vi "T90 Zustandsautomat.vi"(0 "Aktion":T1, 11 "error in (no error)":errorcluster caption="Fehler (Eingang, kein Fehler)") -> (4 "Aktion":T1, 8 "Aufschaltzeit":dbl, 10 "Status":string, 15 "error out":errorcluster caption="Fehler (Ausgang)")   [LabVIEW 2020, in "EPA 1065.lvlib" / "T90 Test 1065-308.lvlib"]
uses:
  T90 Test 1065-308.lvlib
  Aktion T90 Zustandsautomat.ctl
  Aktion FGV Datenmanagment.ctl
  Sprachverwaltung/FGV Aktion Tabelle zerlegen.ctl
  Aktion FGV T90.ctl
  Seiten/CalGas Aufschaltung/FGV CalGas Aktionen.ctl
  Seiten/CalGas Aufschaltung/Auswahl Aufschaltpunkt.ctl
  Funktionstasten/Zustaende.ctl
  Funktionstasten/Funktionstasten-Aktion.ctl
  PNS/Aktionen FGV Grenzwerte.ctl
  Sprachverwaltung/Sprachverwaltung.lvlib
  Funktionstasten/Funktionstasten.lvlib
  Allgemein/allgemeine Sub-VIs.lvlib
  Seiten/CalGas Aufschaltung/CalGas Aufschaltung.lvlib
  PNS/PNS.lvlib
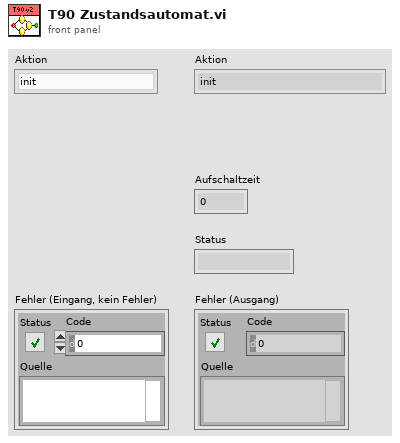
[diagram p1: front panel]
types:
  T1 = typedef "EPA 1065.lvlib/T90 Test 1065-308.lvlib/Aktion T90 Zustandsautomat.ctl" = enum16{"init", "start", "CG aufschalten", "Aufschaltzeit einhalten", "Peak ermitteln", "spülen", "CG Sequenz T10", "CG Sequenz T90", "CG halten", "N2 Sequenz T90", "N2 Sequenz T10", "N2 halten", "Auswerten", "abbrechen", "Störung", "fertig"}
  T2 = typedef "EPA 1065.lvlib/T90 Test 1065-308.lvlib/Aktion FGV Datenmanagment.ctl" = enum16{"init", "lesen", "Istwerte schreiben", "höchsten Peak setzen", "Auswerten", "Grenzen setzen", "Sollwert ändern", "Rise T10", "Rise T90", "Fall T90", "Fall T10", "Bit löschen", "Umschaltzeitpunkt"}
  T3 = typedef "Sprachverwaltung.lvlib/FGV Aktion Tabelle zerlegen.ctl" = enum16{"laden", "vereinzeln", "speichern"}
  T4 = typedef "CalGas Aufschaltung.lvlib/FGV CalGas Aktionen.ctl" = enum16{"lesen", "Analysator Auswahl", "Def.CalGas", "Aufschaltung CalGas", "laden", "speichern", "KAL extrahieren"}
  T5 = typedef "EPA 1065.lvlib/T90 Test 1065-308.lvlib/Aktion FGV T90.ctl" = enum16{"lesen", "Konfig Daten", "speichern", "laden", "T90 aktiv", "T90 inaktiv", "Ext. Ventil aktivieren", "Ext. Ventil deaktivieren", "N2 spülen aktiv", "N2 spülen inaktiv", "Ergebnis Textfile"}
  T6 = typedef "CalGas Aufschaltung.lvlib/Auswahl Aufschaltpunkt.ctl" = enum16{"über Filterblock", "Analysator direkt", "über PNS", "Entnahme", "Gasdivider"}
  T7 = typedef "Funktionstasten.lvlib/Funktionstasten-Aktion.ctl" = enum16{"Initialisieren", "Zustand setzen", "Taste gedrückt", "Fehler speichern", "Lesen", "Manuell", "Remote", "Bitparallel", "Samplepoint", "Zeit Prüfen", "reset Umschalten"}
  T8 = typedef "Funktionstasten.lvlib/Zustaende.ctl" = enum16{"Standby", "Pause", "Eco", "Messen", "Kalibrieren", "Spülen Filter", "Spülen Leitung", "Umgebungsluft", "0-Gas", "Cal-Gas", "CG zu PNS", "-------------", "Init 1", "Init 2", "Init 3", "Init 4", "Messen vorbereiten", "Messen durchführen", "Exit"}
  T9 = typedef "PNS.lvlib/Aktionen FGV Grenzwerte.ctl" = enum16{"lesen", "Grenzw. schreiben", "Anweisungscode", "IP-Adresse", "laden", "speichern", "Anweisungscode vorgeben"}
  T10 = typedef "CalGas Aufschaltung.lvlib/Aufschaltung CalGas.ctl" = cluster{"Kalibriergas":T11, "Aufschaltpunkt":T6, "Analysator":T12}
  T11 = typedef "Auswahlfeld.ctl" = u16
  T12 = typedef "CalGas Aufschaltung.lvlib/Auswahl Analysator.ctl" = enum16{"FT-IR", "FID", "PMA", "PMA/FID/FT-IR"}
  T13 = typedef "EPA 1065.lvlib/T90 Test 1065-308.lvlib/T90 Konfig Daten.ctl" = cluster{"Bearbeiter:":string, "Komponente:":u16, "Gasflaschen Nr.:":string, "Accuracy":dbl, "Sollwert":dbl, "Modus":T14, "Abschaltzeit:":dbl, "Abweichung:":dbl, "Pfad:":path, "Textname:":string, "CG Aufschaltzeit:":dbl, "Einheit":string, "N2 Aufschaltzeit:":dbl, "Analysator":T15, "Gasflasche":T16, "Konfig Gasflasche":T17, "Frequency:":T18}
  T14 = typedef "EPA 1065.lvlib/T90 Test 1065-308.lvlib/Modus.ctl" = u16
  T15 = typedef "System Einstellungen V2.lvlib/Analysatoren.ctl" = string
  T16 = typedef "System Einstellungen V2.lvlib/Gasflasche Auswahl.ctl" = u16
  T17 = typedef "System Einstellungen V2.lvlib/Konfig Gasflasche.ctl" = bool
  T18 = typedef "EPA 1065.lvlib/T90 Test 1065-308.lvlib/Frequenz.ctl" = u16
  T19 = typedef "EPA 1065.lvlib/T90 Test 1065-308.lvlib/Datencluster.ctl" = cluster{"Höchster Peak":T20, "T10 Grenzwert":T20, "T90 Grenzwert":T20, "Rise Times":dbl[], "Fall Times":dbl[], "RiseTime gemittelt":T20, "FallTime gemittelt":T20, "Zeitstempel":timestamp[], "Rise T10":bool, "Rise T90":bool, "Fall T10":bool, "Fall T90":bool, "RiseTime >5":bool, "Falltime >5":bool, "RiseTime <10":bool, "Falltime <10":bool, "T0-T90":dbl[], "T100-T10":dbl[]}
  T20 = typedef "Zahlen-Eingabefeld.ctl" = sgl
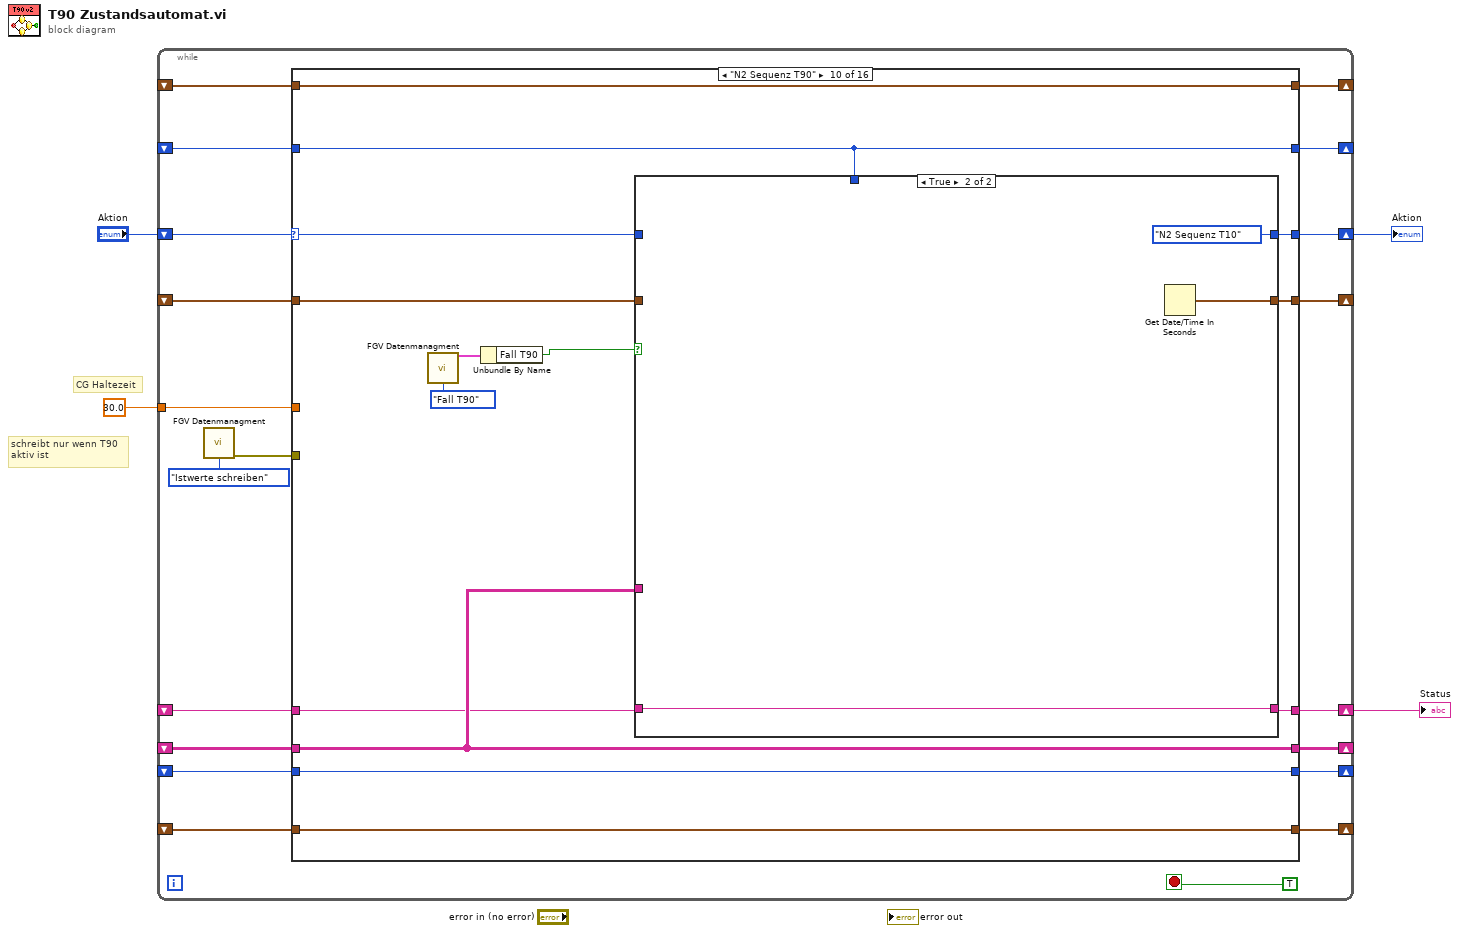
[diagram p0: block diagram]
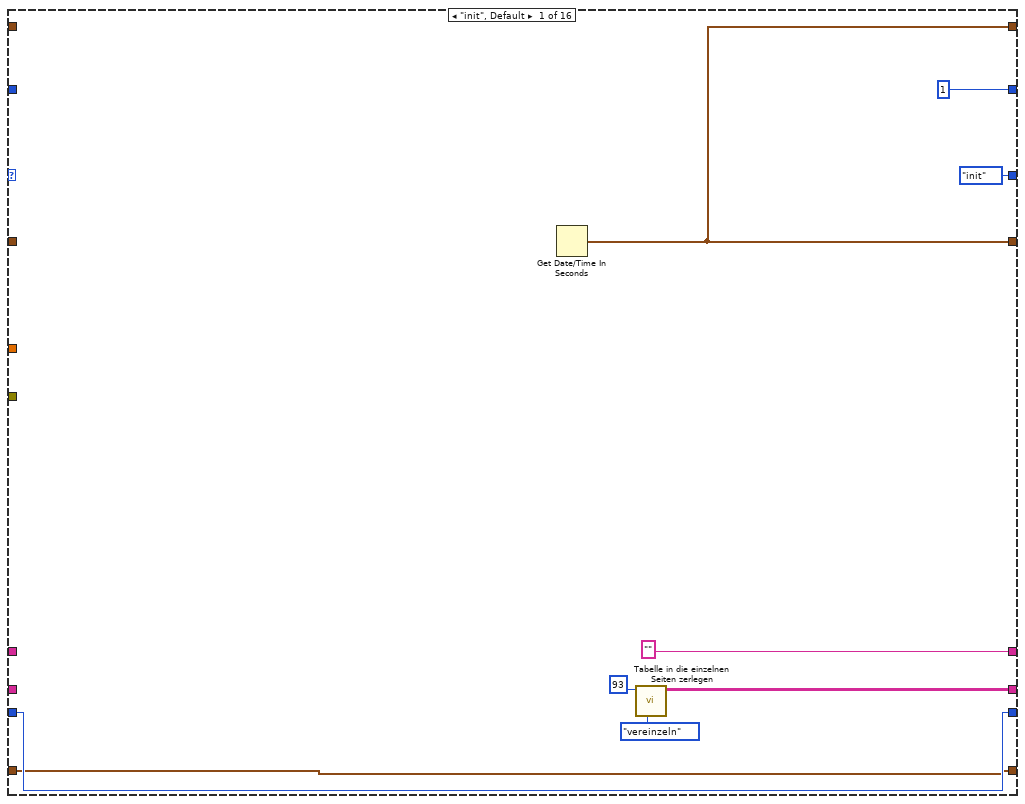
[diagram p2: hidden frame]
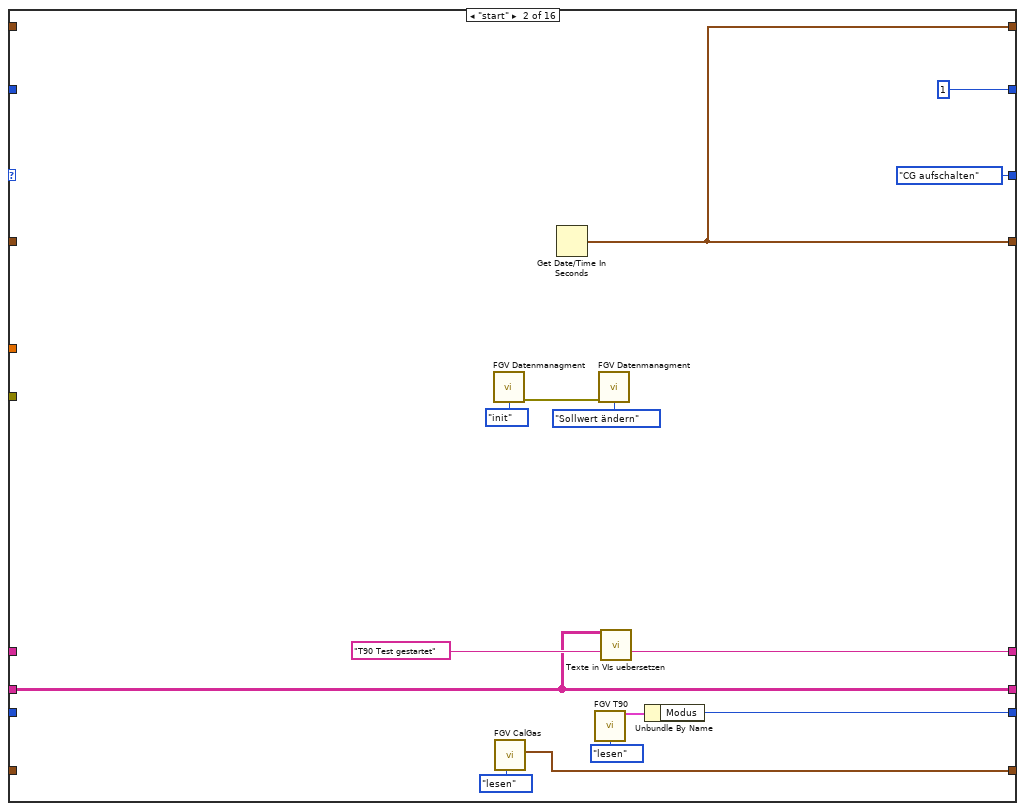
[diagram p3: hidden frame]
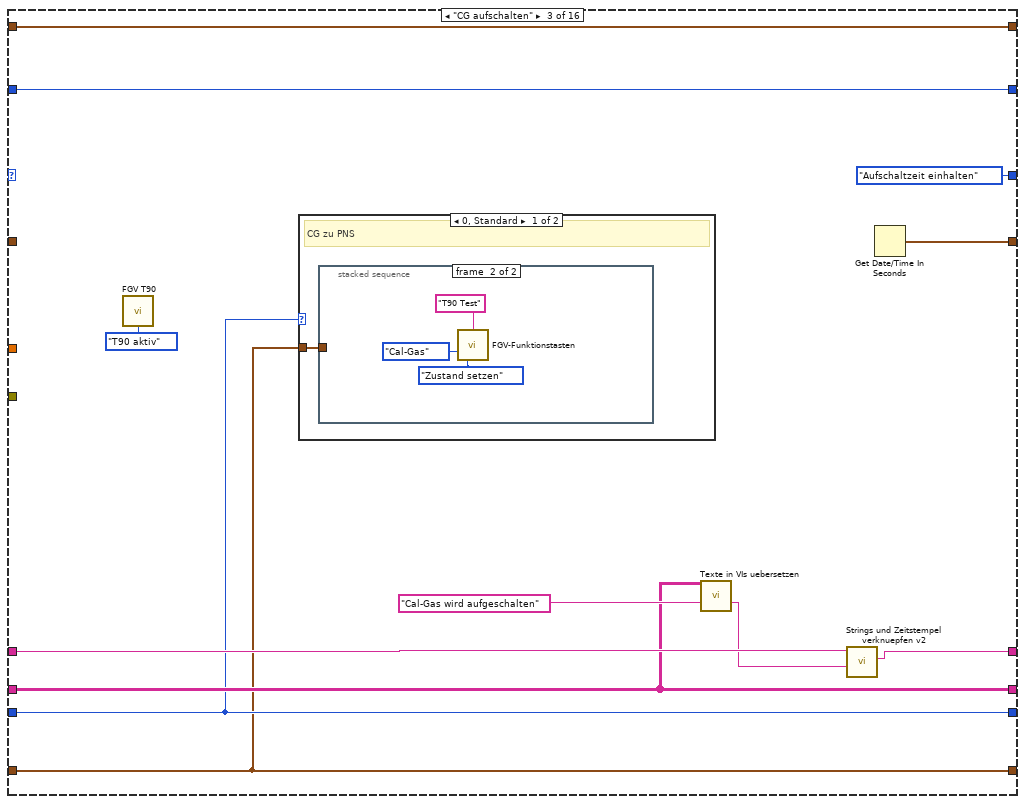
[diagram p4: hidden frame]
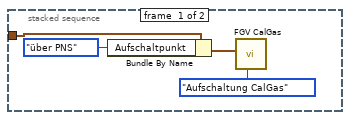
[diagram p5: hidden frame]
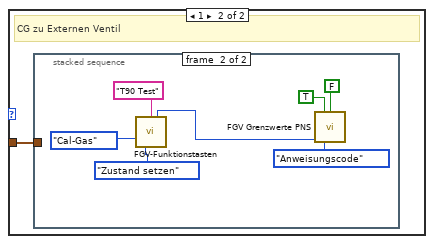
[diagram p6: hidden frame]
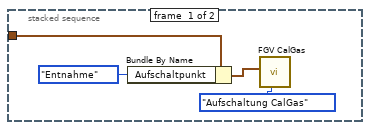
[diagram p7: hidden frame]
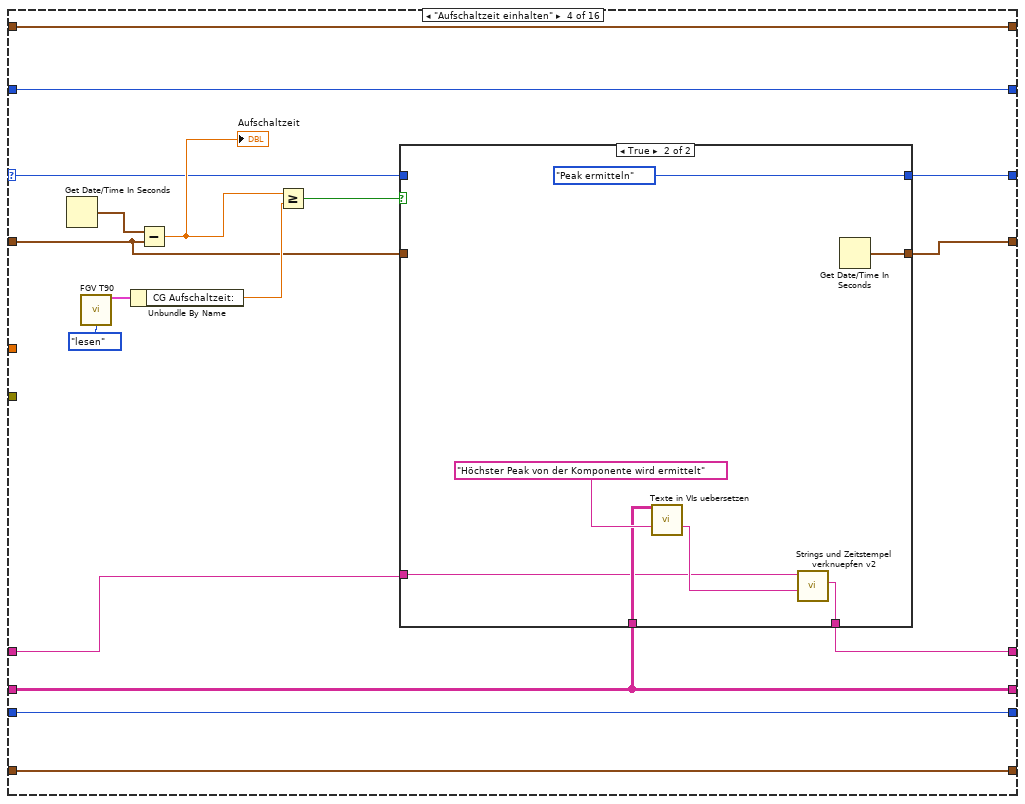
[diagram p8: hidden frame]
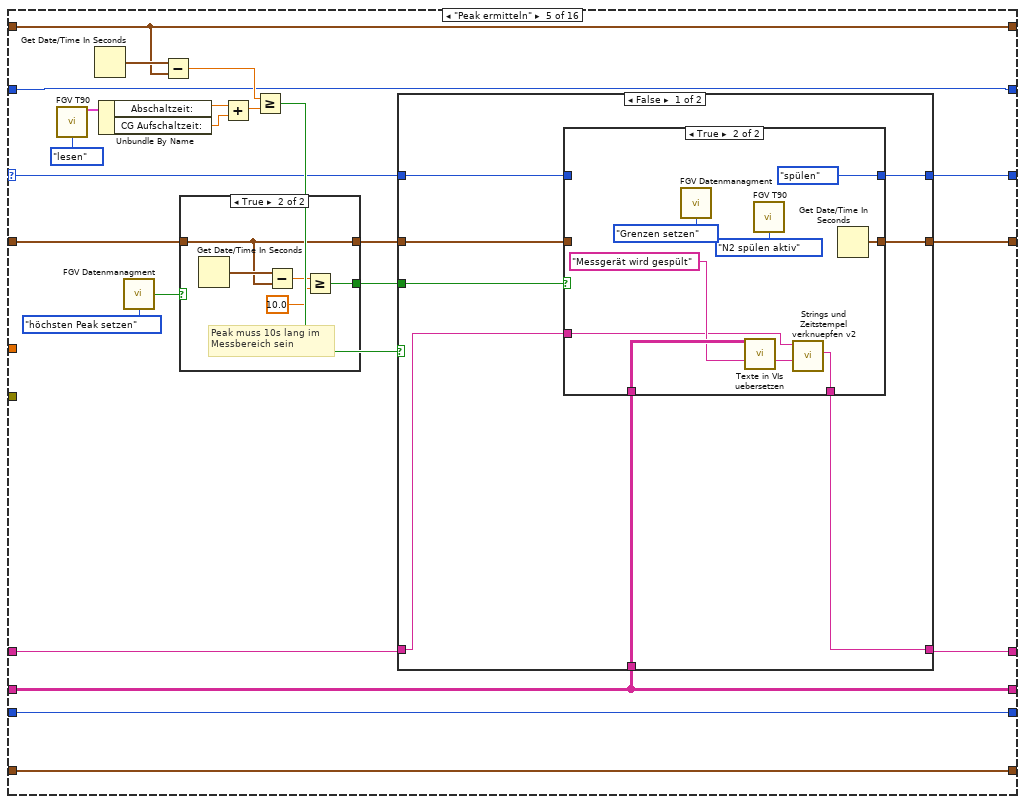
[diagram p10: hidden frame]
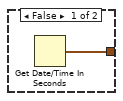
[diagram p11: hidden frame]
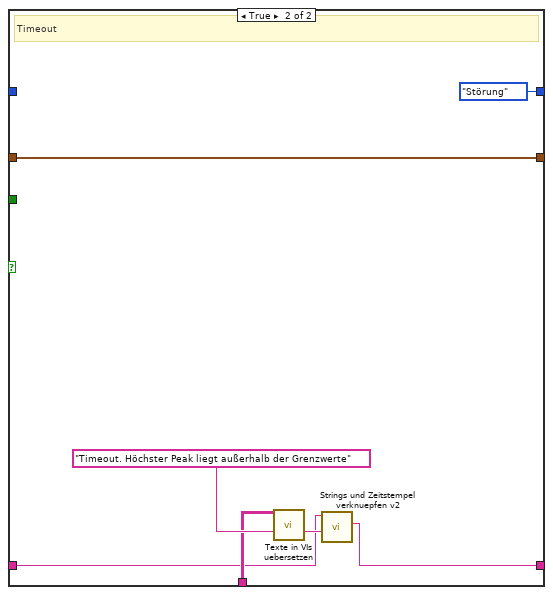
[diagram p13: hidden frame]
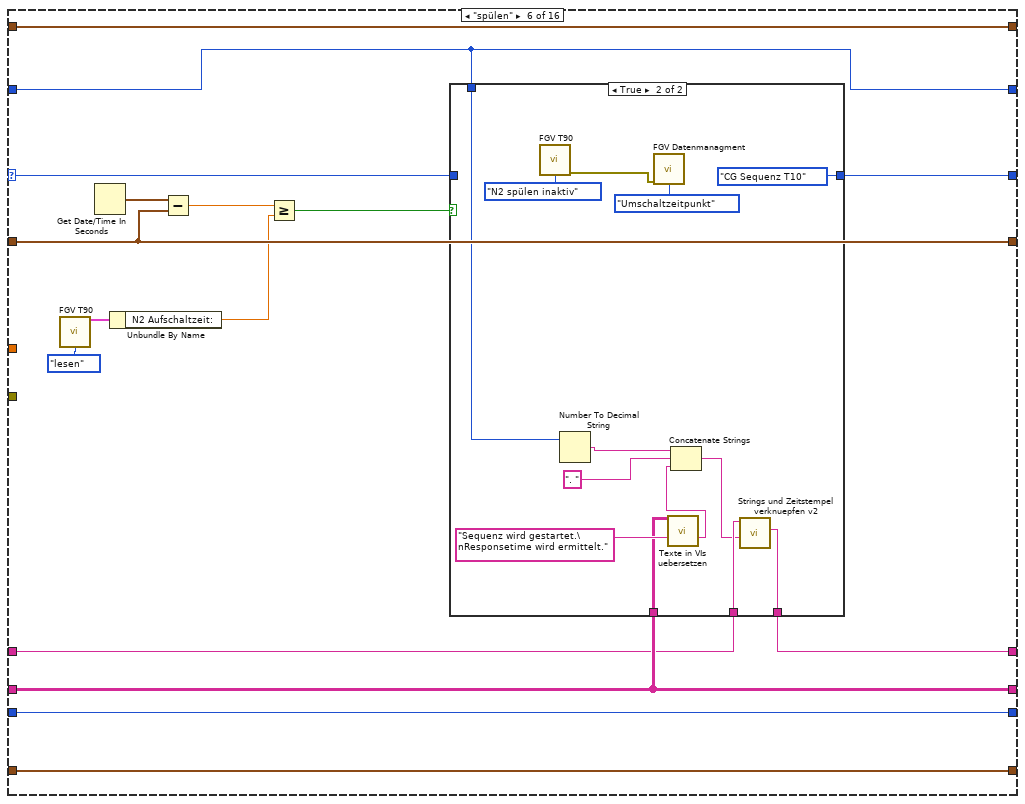
[diagram p14: hidden frame]
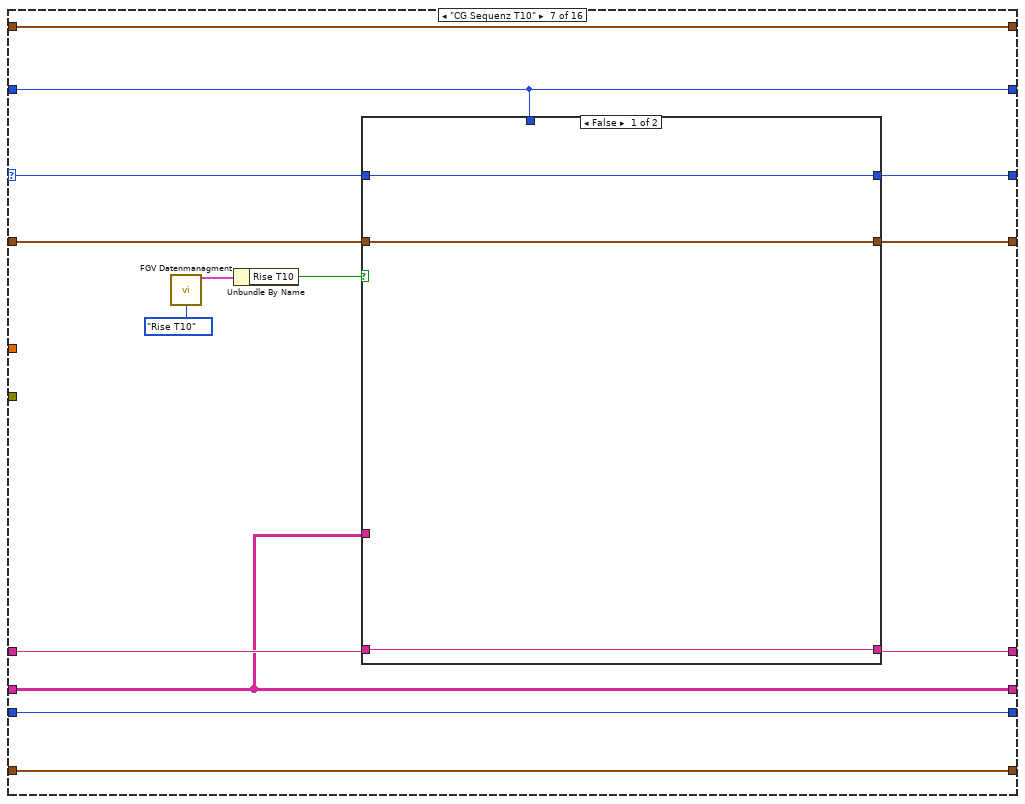
[diagram p16: hidden frame]
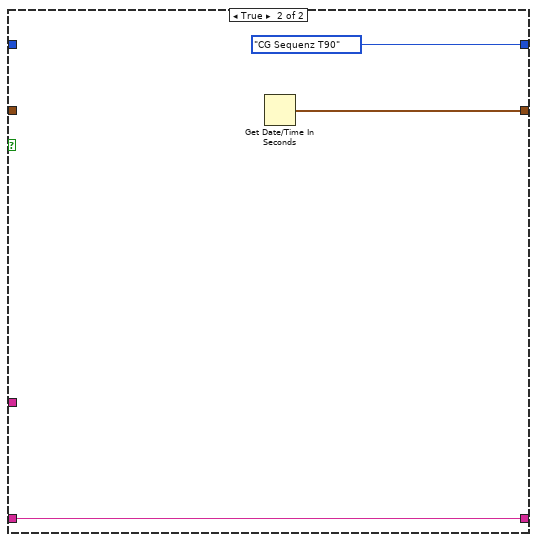
[diagram p17: hidden frame]
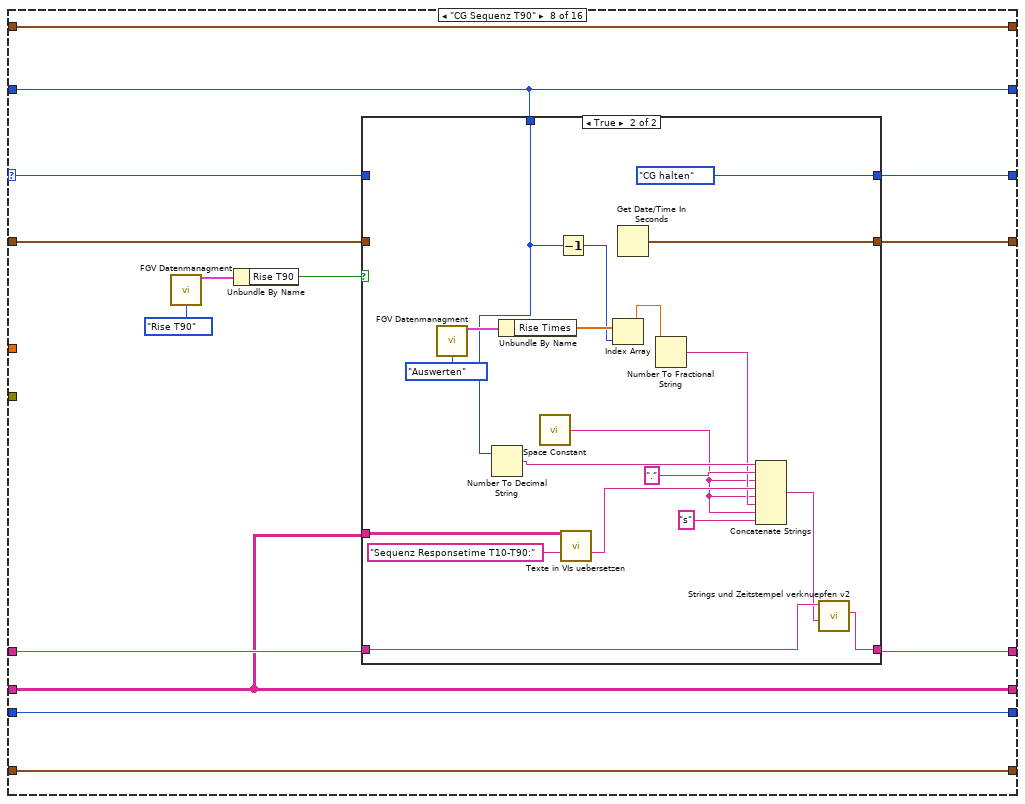
[diagram p18: hidden frame]
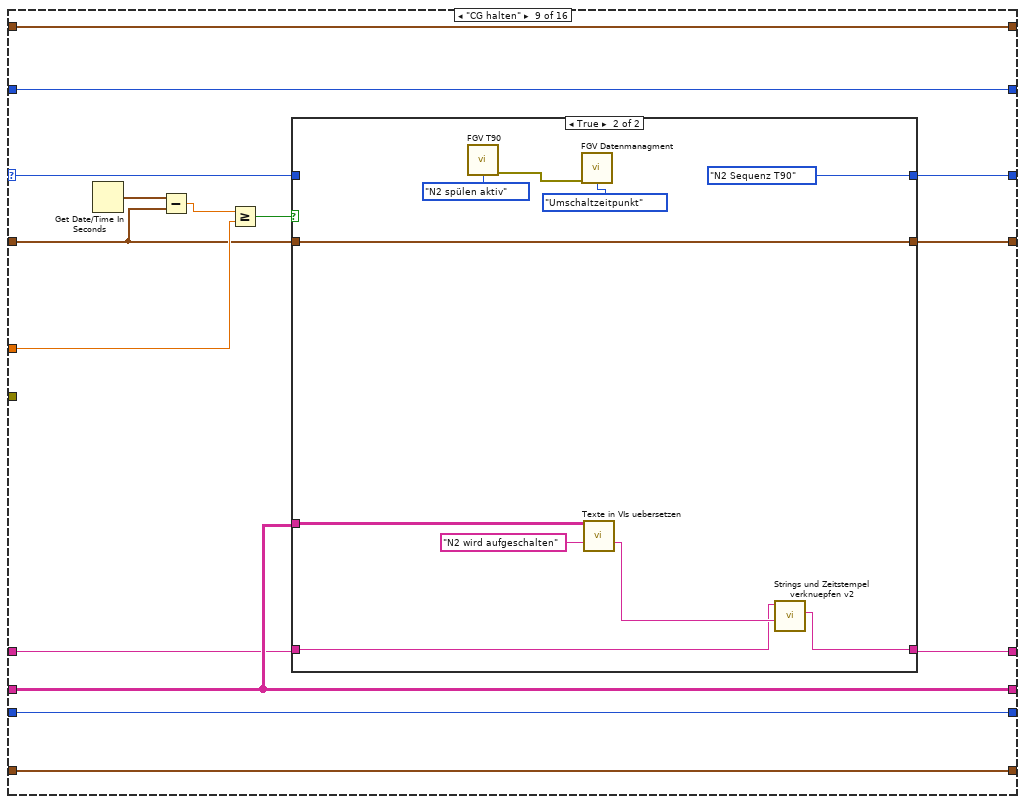
[diagram p20: hidden frame]
diagram:
  # "schreibt nur wenn T90\naktiv ist"
  # "CG Haltezeit"
  n1 = while {
    shift-right: [w23] -> w1
    shift-left: "Aktion" -> [w22]
    shift-right: [w21] -> _
    shift-left: _ -> [w20]
    shift-right: [w19] -> w3
    shift-left: _ -> [w17]
    shift-right: [w16] -> _
    shift-left: _ -> [w18]
    tunnel: 30.0 ("x-y") -> [w15]
    shift-right: [w14] -> _
    shift-left: _ -> [w13]
    shift-right: [w11] -> _
    shift-left: _ -> [w12]
    shift-right: [w8] -> _
    shift-left: _ -> [w7]
    shift-right: [w6] -> _
    shift-left: _ -> [w5]
    stop <- TRUE stop-if-true
    n2 = call "FGV Datenmanagment.vi"("Aktion"=Aktion_FGV_Datenmanagment."Istwerte schreiben") -> ("error out"=w9:errorcluster)  [unwired: 7 in, 7 out]
    n3 = case shown="\"N2 Sequenz T90\"" w22 {
      selector: w22 -> [_ _ _ w89 w122 w174 w205 w225 w260 w289 w309 w349 _ _ _ _]
      tunnel: [Aktion_T90_Zustandsautomat."init" ("Aktion") Aktion_T90_Zustandsautomat."CG aufschalten" ("Aktion") Aktion_T90_Zustandsautomat."Aufschaltzeit einhalten" ("Aktion") w91 w123 w173 w204 w224 w259 w288 w308 w348 Aktion_T90_Zustandsautomat."fertig" ("Aktion") Aktion_T90_Zustandsautomat."fertig" ("Aktion") Aktion_T90_Zustandsautomat."fertig" ("Aktion") Aktion_T90_Zustandsautomat."fertig" ("Aktion")] -> w23
      tunnel: [w27 w44 w59 w82 w117 w177 w203 w223 w257 w287 w307 w346 w387 w406 w418 w426] -> w16
      tunnel: [w30 w40 w52 w87 w120 w172 w199 w219 w255 w285 w305 w343 w394 w404 w422 w430] -> w21
      tunnel: w20 -> [_ w40 w52 w87 w120 w172 w199 w219 w255 w285 w305 w343 w394 w404 w422 w430]
      tunnel: ["" w34 w55 w86 w118 w170 w200 w220 w253 w284 w304 w341 w385 w395 w416 w425] -> w19
      tunnel: w18 -> [_ _ _ w83 w111 w177 w202 w222 w258 w286 w306 w347 w387 w406 w418 w426]
      tunnel: w17 -> [_ _ w56 w85 w119 w171 w201 w221 w254 w283 w303 w342 w385 _ w416 w425]
      tunnel: w15 -> [_ _ _ _ _ _ _ _ w262 _ _ _ _ _ _ _]
      tunnel: [1 1 w57 w88 w121 w169 w198 w218 w256 w282 w302 w344 w393 w408 w419 w429] -> w14
      tunnel: w13 -> [_ _ w57 w88 w121 w169 w198 w218 w256 w282 w302 w345 w393 w408 w419 w429]
      tunnel: [w27 w44 w51 w84 w116 w168 w197 w217 w252 w281 w301 w340 w384 w403 w417 w428] -> w11
      tunnel: w12 -> [_ _ w51 w84 w116 w168 w197 w217 w252 w281 w301 w340 w384 w403 w417 w428]
      tunnel: w9 -> [_ _ _ _ _ _ _ _ _ _ _ _ _ _ _ _]
      tunnel: [w26 w37 w49 w81 w108 w167 w195 w215 w251 w279 w299 w339 w383 w398 w411 w424] -> w8
      tunnel: w7 -> [w26 _ w49 w81 w108 w167 w195 w215 w251 w279 w299 w339 w383 w398 w411 w424]
      tunnel: [w25 w35 w48 w80 w107 w166 w194 w214 w250 w278 w298 w338 w381 w396 w409 w423] -> w6
      tunnel: w5 -> [w25 _ w48 w80 w107 w166 w194 w214 w250 w278 w298 w338 w381 w396 w409 w423]
      frame "init", Default {
        n4 = Get Date/Time In Seconds() -> (seconds since 1Jan1904=w27:timestamp)
        n5 = call "Tabelle in die einzelnen Seiten zerlegen.vi"("Aktion"=FGV_Aktion_Tabelle_zerlegen."vereinzeln", "Index (Seite)"=93) -> ("Sprachliste"=w30:string[][])  [unwired: 7 in, 2 out]
      }
      frame "start" {
        n6 = call "FGV Datenmanagment.vi"("Aktion"=Aktion_FGV_Datenmanagment."init") -> ("error out"=w42:errorcluster)  [unwired: 7 in, 7 out]
        n7 = call "FGV CalGas.vi"("Aktionen"=FGV_CalGas_Aktionen."lesen") -> ("Aufschaltung CalGas"=w35:T10)  [unwired: 6 in, 4 out]
        n8 = Get Date/Time In Seconds() -> (seconds since 1Jan1904=w44:timestamp)
        n9 = call "FGV T90.vi"("Aktion"=Aktion_FGV_T90."lesen") -> ("T90 Konfig Daten"=w38:T13)  [unwired: 9 in, 5 out]
        n10 = call "FGV Datenmanagment.vi"("error in (no error)"=w42, "Aktion"=Aktion_FGV_Datenmanagment."Sollwert ändern") -> ()  [unwired: 6 in, 8 out]
        n11 = call "Texte in VIs uebersetzen.vi"("Sprachliste"=w40, "String zum Übersetzen"="T90 Test gestartet" ("String 1 hinzufügen")) -> ("String zum Übersetzen"=w34:string)  [unwired: 9 in, 4 out]
        n12 = Unbundle By Name(w38) -> ("Modus"=w37:T14)
      }
      frame "CG aufschalten" {
        n13 = call "FGV T90.vi"("Aktion"=Aktion_FGV_T90."T90 aktiv") -> ()  [unwired: 9 in, 6 out]
        n14 = case shown="0, Standard" w49 {
          tunnel: w48 -> [w60 w68]
          frame 0, Default {
            # "CG zu PNS"
            n15 = stacked-sequence {
              tunnel: w60 -> [w63 _]
              frame #0 {
                n16 = Bundle By Name(cluster=w63, "Aufschaltpunkt"=Auswahl_Aufschaltpunkt."über PNS") -> (w61:T10)
                n17 = call "FGV CalGas.vi"("Aktionen"=FGV_CalGas_Aktionen."Aufschaltung CalGas", "Aufschaltung CalGas"=w61) -> ()  [unwired: 5 in, 5 out]
              }
              frame #1 {
                n18 = call "FGV-Funktionstasten.vi"("Herkunft"="T90 Test", "Zustand"=Zustaende."Cal-Gas", "Aktion"=Funktionstasten-Aktion."Zustand setzen") -> ()  [unwired: 5 in, 8 out]
              }
            }
          }
          frame 1 {
            # "CG zu Externen Ventil"
            n19 = stacked-sequence {
              tunnel: w68 -> [w71 _]
              frame #0 {
                n20 = Bundle By Name(cluster=w71, "Aufschaltpunkt"=Auswahl_Aufschaltpunkt."Entnahme") -> (w70:T10)
                n21 = call "FGV CalGas.vi"("Aktionen"=FGV_CalGas_Aktionen."Aufschaltung CalGas", "Aufschaltung CalGas"=w70) -> ()  [unwired: 5 in, 5 out]
              }
              frame #1 {
                n22 = call "FGV-Funktionstasten.vi"("Herkunft"="T90 Test", "Zustand"=Zustaende."Cal-Gas", "Aktion"=Funktionstasten-Aktion."Zustand setzen") -> ("Samplepoint"=w73:u16)  [unwired: 5 in, 7 out]
                n23 = call "FGV Grenzwerte PNS.vi"("T90"=TRUE ("T90 lüften"), "T90 lüften"=FALSE, "Samplepoint"=w73, "Aktionen FGV Grenzwerte"=Aktionen_FGV_Grenzwerte."Anweisungscode") -> ()  [unwired: 9 in, 3 out]
              }
            }
          }
        }
        n24 = call "Texte in VIs uebersetzen.vi"("Sprachliste"=w52, "String zum Übersetzen"="Cal-Gas wird aufgeschalten" ("String 1 hinzufügen")) -> ("String zum Übersetzen"=w53:string)  [unwired: 9 in, 4 out]
        n25 = call "Strings und Zeitstempel verknuepfen v2.vi"("String 1 hinzufügen"=w53, "Eingangs String"=w56) -> ("Verknüpfter String"=w55:string)  [unwired: 9 in]
        n26 = Get Date/Time In Seconds() -> (seconds since 1Jan1904=w59:timestamp)
      }
      frame "Aufschaltzeit einhalten" {
        n27 = Get Date/Time In Seconds() -> (seconds since 1Jan1904=w96:timestamp)
        n28 = call "FGV T90.vi"("Aktion"=Aktion_FGV_T90."lesen") -> ("T90 Konfig Daten"=w94:T13)  [unwired: 9 in, 5 out]
        n29 = Unbundle By Name(w94) -> ("CG Aufschaltzeit:"=w92:dbl)
        n30 = Subtract(x=w96, y=w83) -> (x-y=w93:dbl)
        "Aufschaltzeit" <- w93
        n31 = Greater Or Equal?(x=w93, y=w92) -> (x >= y?=w90:bool)
        n32 = case shown="True" w90 {
          tunnel: [w99 Aktion_T90_Zustandsautomat."Peak ermitteln" ("Aktion")] -> w91
          tunnel: w89 -> [w99 _]
          tunnel: w87 -> [_ w103]
          tunnel: [w98 w102] -> w86
          tunnel: w85 -> [w98 w101]
          tunnel: w83 -> [w97 _]
          tunnel: [w97 w100] -> w82
          frame False {
          }
          frame True {
            n33 = call "Texte in VIs uebersetzen.vi"("Sprachliste"=w103, "String zum Übersetzen"="Höchster Peak von der Komponente wird ermittelt" ("String 1 hinzufügen")) -> ("String zum Übersetzen"=w104:string)  [unwired: 9 in, 4 out]
            n34 = call "Strings und Zeitstempel verknuepfen v2.vi"("String 1 hinzufügen"=w104, "Eingangs String"=w101) -> ("Verknüpfter String"=w102:string)  [unwired: 9 in]
            n35 = Get Date/Time In Seconds() -> (seconds since 1Jan1904=w100:timestamp)
          }
        }
      }
      frame "Peak ermitteln" {
        n36 = call "FGV T90.vi"("Aktion"=Aktion_FGV_T90."lesen") -> ("T90 Konfig Daten"=w127:T13)  [unwired: 9 in, 5 out]
        n37 = Get Date/Time In Seconds() -> (seconds since 1Jan1904=w129:timestamp)
        n38 = Unbundle By Name(w127) -> ("Abschaltzeit:"=w125:dbl, "CG Aufschaltzeit:"=w114:dbl)
        n39 = call "FGV Datenmanagment.vi"("Aktion"=Aktion_FGV_Datenmanagment."höchsten Peak setzen") -> ("Peak im Bereich"=w112:bool)  [unwired: 7 in, 7 out]
        n40 = Subtract(x=w129, y=w116) -> (x-y=w124:dbl)
        n41 = case shown="True" w112 {
          tunnel: w111 -> [_ w134]
          tunnel: [w130 w134] -> w110
          tunnel: [_ w131] -> w109
          frame False {
            n42 = Get Date/Time In Seconds() -> (seconds since 1Jan1904=w130:timestamp)
          }
          frame True {
            # "Peak muss 10s lang im \nMessbereich sein"
            n43 = Get Date/Time In Seconds() -> (seconds since 1Jan1904=w135:timestamp)
            n44 = Subtract(x=w135, y=w134) -> (x-y=w133:dbl)
            n45 = Greater Or Equal?(x=w133, y=10.0) -> (x >= y?=w131:bool)
          }
        }
        n46 = Add(x=w125, y=w114) -> (x+y=w115:dbl)
        n47 = Greater Or Equal?(x=w124, y=w115) -> (x >= y?=w126:bool)
        n48 = case shown="False" w126 {
          tunnel: [w143 Aktion_T90_Zustandsautomat."Störung" ("Aktion")] -> w123
          tunnel: w122 -> [w142 _]
          tunnel: w120 -> [w141 w159]
          tunnel: w119 -> [w140 w158]
          tunnel: [w139 w157] -> w118
          tunnel: w110 -> [w137 w156]
          tunnel: [w138 w156] -> w117
          tunnel: w109 -> [w136 _]
          frame False {
            n49 = case shown="True" w136 {
              tunnel: [w146 Aktion_T90_Zustandsautomat."spülen" ("Aktion")] -> w143
              tunnel: w142 -> [w146 _]
              tunnel: w141 -> [_ w152]
              tunnel: w140 -> [w145 w150]
              tunnel: [w145 w149] -> w139
              tunnel: [w144 w147] -> w138
              tunnel: w137 -> [w144 _]
              frame False {
              }
              frame True {
                n50 = call "FGV Datenmanagment.vi"("Aktion"=Aktion_FGV_Datenmanagment."Grenzen setzen") -> ()  [unwired: 7 in, 8 out]
                n51 = call "Texte in VIs uebersetzen.vi"("Sprachliste"=w152, "String zum Übersetzen"="Messgerät wird gespült") -> ("String zum Übersetzen"=w153:string)  [unwired: 9 in, 4 out]
                n52 = call "FGV T90.vi"("Aktion"=Aktion_FGV_T90."N2 spülen aktiv") -> ()  [unwired: 9 in, 6 out]
                n53 = call "Strings und Zeitstempel verknuepfen v2.vi"("String 1 hinzufügen"=w153, "Eingangs String"=w150) -> ("Verknüpfter String"=w149:string)  [unwired: 9 in]
                n54 = Get Date/Time In Seconds() -> (seconds since 1Jan1904=w147:timestamp)
              }
            }
          }
          frame True {
            # "Timeout"
            n55 = call "Texte in VIs uebersetzen.vi"("Sprachliste"=w159, "String zum Übersetzen"="Timeout. Höchster Peak liegt außerhalb der Grenzwerte") -> ("String zum Übersetzen"=w161:string)  [unwired: 9 in, 4 out]
            n56 = call "Strings und Zeitstempel verknuepfen v2.vi"("String 1 hinzufügen"=w161, "Eingangs String"=w158) -> ("Verknüpfter String"=w157:string)  [unwired: 9 in]
          }
        }
      }
      frame "spülen" {
        n57 = call "FGV T90.vi"("Aktion"=Aktion_FGV_T90."lesen") -> ("T90 Konfig Daten"=w164:T13)  [unwired: 9 in, 5 out]
        n58 = Get Date/Time In Seconds() -> (seconds since 1Jan1904=w178:timestamp)
        n59 = Unbundle By Name(w164) -> ("N2 Aufschaltzeit:"=w163:dbl)
        n60 = Subtract(x=w178, y=w177) -> (x-y=w176:dbl)
        n61 = Greater Or Equal?(x=w176, y=w163) -> (x >= y?=w175:bool)
        n62 = case shown="True" w175 {
          tunnel: w174 -> [w180 _]
          tunnel: [w180 Aktion_T90_Zustandsautomat."CG Sequenz T10" ("Aktion")] -> w173
          tunnel: w172 -> [_ w190]
          tunnel: w171 -> [w179 w189]
          tunnel: [w179 w188] -> w170
          tunnel: w169 -> [_ w187]
          frame False {
          }
          frame True {
            n63 = call "FGV T90.vi"("Aktion"=Aktion_FGV_T90."N2 spülen inaktiv") -> ("error out"=w181:errorcluster)  [unwired: 9 in, 5 out]
            n64 = Number To Decimal String(number=w187) -> (decimal integer string=w186:string)  [unwired: 1 in]
            n65 = call "FGV Datenmanagment.vi"("error in (no error)"=w181, "Aktion"=Aktion_FGV_Datenmanagment."Umschaltzeitpunkt") -> ()  [unwired: 6 in, 8 out]
            n66 = call "Texte in VIs uebersetzen.vi"("Sprachliste"=w190, "String zum Übersetzen"="Sequenz wird gestartet.\nResponsetime wird ermittelt.") -> ("String zum Übersetzen"=w184:string)  [unwired: 9 in, 4 out]
            n67 = Concatenate Strings(w186, ". ", w184) -> (w183:string)
            n68 = call "Strings und Zeitstempel verknuepfen v2.vi"("String 1 hinzufügen"=w183, "Eingangs String"=w189) -> ("Verknüpfter String"=w188:string)  [unwired: 9 in]
          }
        }
      }
      frame "CG Sequenz T10" {
        n69 = call "FGV Datenmanagment.vi"("Aktion"=Aktion_FGV_Datenmanagment."Rise T10") -> ("Daten"=w196:T19)  [unwired: 7 in, 7 out]
        n70 = Unbundle By Name(w196) -> ("Rise T10"=w206:bool)
        n71 = case shown="False" w206 {
          tunnel: w205 -> [w210 _]
          tunnel: [w210 Aktion_T90_Zustandsautomat."CG Sequenz T90" ("Aktion")] -> w204
          tunnel: [w209 w212] -> w203
          tunnel: w202 -> [w209 _]
          tunnel: w201 -> [w208 w211]
          tunnel: [w208 w211] -> w200
          tunnel: w199 -> [_ _]
          tunnel: w198 -> [_ _]
          frame False {
          }
          frame True {
            n72 = Get Date/Time In Seconds() -> (seconds since 1Jan1904=w212:timestamp)
          }
        }
      }
      frame "CG Sequenz T90" {
        n73 = call "FGV Datenmanagment.vi"("Aktion"=Aktion_FGV_Datenmanagment."Rise T90") -> ("Daten"=w216:T19)  [unwired: 7 in, 7 out]
        n74 = Unbundle By Name(w216) -> ("Rise T90"=w226:bool)
        n75 = case shown="True" w226 {
          tunnel: w225 -> [w230 _]
          tunnel: [w230 Aktion_T90_Zustandsautomat."CG halten" ("Aktion")] -> w224
          tunnel: [w229 w248] -> w223
          tunnel: w222 -> [w229 _]
          tunnel: w221 -> [w228 w247]
          tunnel: [w228 w246] -> w220
          tunnel: w219 -> [_ w232]
          tunnel: w218 -> [_ w238]
          frame False {
          }
          frame True {
            n76 = call "FGV Datenmanagment.vi"("Aktion"=Aktion_FGV_Datenmanagment."Auswerten") -> ("Daten"=w244:T19)  [unwired: 7 in, 7 out]
            n77 = Number To Decimal String(number=w238) -> (decimal integer string=w240:string)  [unwired: 1 in]
            n78 = Unbundle By Name(w244) -> ("Rise Times"=w243:dbl[])
            n79 = call <vilib>:"Space Constant.vi"() -> ("String"=w234:string)
            n80 = Decrement(x=w238) -> (x-1=w242:i32)
            n81 = call "Texte in VIs uebersetzen.vi"("Sprachliste"=w232, "String zum Übersetzen"="Sequenz Responsetime T10-T90:") -> ("String zum Übersetzen"=w236:string)  [unwired: 9 in, 4 out]
            n82 = Index Array(array=w243, index=w242) -> (element=w241:dbl)
            n83 = Get Date/Time In Seconds() -> (seconds since 1Jan1904=w248:timestamp)
            n84 = Number To Fractional String(number=w241) -> (F-format string=w235:string)  [unwired: 3 in]
            n85 = Concatenate Strings(w240, ".", w234, w236, w234, w235, w234, "s" ("String")) -> (w231:string)
            n86 = call "Strings und Zeitstempel verknuepfen v2.vi"("String 1 hinzufügen"=w231, "Eingangs String"=w247) -> ("Verknüpfter String"=w246:string)  [unwired: 9 in]
          }
        }
      }
      frame "CG halten" {
        n87 = Get Date/Time In Seconds() -> (seconds since 1Jan1904=w264:timestamp)
        n88 = Subtract(x=w264, y=w258) -> (x-y=w263:dbl)
        n89 = Greater Or Equal?(x=w263, y=w262) -> (x >= y?=w261:bool)
        n90 = case shown="True" w261 {
          tunnel: w260 -> [w267 _]
          tunnel: [w267 Aktion_T90_Zustandsautomat."N2 Sequenz T90" ("Aktion")] -> w259
          tunnel: w258 -> [w266 w275]
          tunnel: [w266 w275] -> w257
          tunnel: w255 -> [_ w273]
          tunnel: w254 -> [w265 w271]
          tunnel: [w265 w270] -> w253
          frame False {
          }
          frame True {
            n91 = call "FGV T90.vi"("Aktion"=Aktion_FGV_T90."N2 spülen aktiv") -> ("error out"=w268:errorcluster)  [unwired: 9 in, 5 out]
            n92 = call "FGV Datenmanagment.vi"("error in (no error)"=w268, "Aktion"=Aktion_FGV_Datenmanagment."Umschaltzeitpunkt") -> ()  [unwired: 6 in, 8 out]
            n93 = call "Texte in VIs uebersetzen.vi"("Sprachliste"=w273, "String zum Übersetzen"="N2 wird aufgeschalten") -> ("String zum Übersetzen"=w272:string)  [unwired: 9 in, 4 out]
            n94 = call "Strings und Zeitstempel verknuepfen v2.vi"("String 1 hinzufügen"=w272, "Eingangs String"=w271) -> ("Verknüpfter String"=w270:string)  [unwired: 9 in]
          }
        }
      }
      frame "N2 Sequenz T90" {
        n95 = call "FGV Datenmanagment.vi"("Aktion"=Aktion_FGV_Datenmanagment."Fall T90") -> ("Daten"=w280:T19)  [unwired: 7 in, 7 out]
        n96 = Unbundle By Name(w280) -> ("Fall T90"=w290:bool)
        n97 = case shown="True" w290 {
          tunnel: w289 -> [w294 _]
          tunnel: [w294 Aktion_T90_Zustandsautomat."N2 Sequenz T10" ("Aktion")] -> w288
          tunnel: [w293 w296] -> w287
          tunnel: w286 -> [w293 _]
          tunnel: w285 -> [_ _]
          tunnel: [w292 w295] -> w284
          tunnel: w283 -> [w292 w295]
          tunnel: w282 -> [_ _]
          frame False {
          }
          frame True {
            n98 = Get Date/Time In Seconds() -> (seconds since 1Jan1904=w296:timestamp)
          }
        }
      }
      frame "N2 Sequenz T10" {
        n99 = call "FGV Datenmanagment.vi"("Aktion"=Aktion_FGV_Datenmanagment."Fall T10") -> ("Daten"=w300:T19)  [unwired: 7 in, 7 out]
        n100 = Unbundle By Name(w300) -> ("Fall T10"=w310:bool)
        n101 = case shown="True" w310 {
          tunnel: w309 -> [w314 _]
          tunnel: [w314 Aktion_T90_Zustandsautomat."N2 halten" ("Aktion")] -> w308
          tunnel: [w313 w333] -> w307
          tunnel: w306 -> [w313 _]
          tunnel: w305 -> [_ w318]
          tunnel: [w312 w317] -> w304
          tunnel: w303 -> [w312 w316]
          tunnel: w302 -> [_ w315]
          frame False {
          }
          frame True {
            n102 = call "FGV Datenmanagment.vi"("Aktion"=Aktion_FGV_Datenmanagment."Auswerten") -> ("Daten"=w330:T19)  [unwired: 7 in, 7 out]
            n103 = Number To Decimal String(number=w315) -> (decimal integer string=w326:string)  [unwired: 1 in]
            n104 = Unbundle By Name(w330) -> ("Fall Times"=w329:dbl[])
            n105 = call <vilib>:"Space Constant.vi"() -> ("String"=w321:string)
            n106 = Decrement(x=w315) -> (x-1=w328:i32)
            n107 = call "Texte in VIs uebersetzen.vi"("Sprachliste"=w318, "String zum Übersetzen"="Sequenz Responsetime T90-T10:") -> ("String zum Übersetzen"=w323:string)  [unwired: 9 in, 4 out]
            n108 = Index Array(array=w329, index=w328) -> (element=w327:dbl)
            n109 = Number To Fractional String(number=w327) -> (F-format string=w322:string)  [unwired: 3 in]
            n110 = call "FGV Datenmanagment.vi"("Aktion"=Aktion_FGV_Datenmanagment."Bit löschen") -> ()  [unwired: 7 in, 8 out]
            n111 = Concatenate Strings(w326, ".", w321, w323, w321, w322, w321, "s" ("String")) -> (w319:string)
            n112 = call "Strings und Zeitstempel verknuepfen v2.vi"("String 1 hinzufügen"=w319, "Eingangs String"=w316) -> ("Verknüpfter String"=w317:string)  [unwired: 9 in]
            n113 = Get Date/Time In Seconds() -> (seconds since 1Jan1904=w333:timestamp)
          }
        }
      }
      frame "N2 halten" {
        n114 = call "FGV T90.vi"("Aktion"=Aktion_FGV_T90."lesen") -> ("T90 Konfig Daten"=w337:T13)  [unwired: 9 in, 5 out]
        n115 = Get Date/Time In Seconds() -> (seconds since 1Jan1904=w352:timestamp)
        n116 = Unbundle By Name(w337) -> ("N2 Aufschaltzeit:"=w335:dbl)
        n117 = Subtract(x=w352, y=w347) -> (x-y=w351:dbl)
        n118 = Greater Or Equal?(x=w351, y=w335) -> (x >= y?=w350:bool)
        n119 = case shown="True" w350 {
          tunnel: w349 -> [w356 _]
          tunnel: [w356 w362] -> w348
          tunnel: w347 -> [w355 w367]
          tunnel: [w355 w367] -> w346
          tunnel: w345 -> [w354 w366]
          tunnel: [w354 w365] -> w344
          tunnel: w343 -> [_ w359]
          tunnel: w342 -> [w353 w358]
          tunnel: [w353 w357] -> w341
          frame False {
          }
          frame True {
            n120 = Increment(x=w366) -> (x+1=w365:i32)
            n121 = Greater Or Equal?(x=w365, y=8) -> (x >= y?=w360:bool)
            n122 = Select(t=Aktion_T90_Zustandsautomat."Auswerten", s=w360, f=Aktion_T90_Zustandsautomat."CG Sequenz T10" ("Aktion")) -> (s? t:f=w362:T1)
            n123 = case shown="False" w360 {
              tunnel: w359 -> [w372 w378]
              tunnel: w358 -> [w368 w376]
              tunnel: [w371 w377] -> w357
              frame False {
                n124 = call "FGV T90.vi"("Aktion"=Aktion_FGV_T90."N2 spülen inaktiv") -> ("error out"=w369:errorcluster)  [unwired: 9 in, 5 out]
                n125 = call "FGV Datenmanagment.vi"("error in (no error)"=w369, "Aktion"=Aktion_FGV_Datenmanagment."Umschaltzeitpunkt") -> ()  [unwired: 6 in, 8 out]
                n126 = call "Texte in VIs uebersetzen.vi"("Sprachliste"=w372, "String zum Übersetzen"="CG wird aufgeschalten") -> ("String zum Übersetzen"=w373:string)  [unwired: 9 in, 4 out]
                n127 = call "Strings und Zeitstempel verknuepfen v2.vi"("String 1 hinzufügen"=w373, "Eingangs String"=w368) -> ("Verknüpfter String"=w371:string)  [unwired: 9 in]
              }
              frame True {
                n128 = call "Texte in VIs uebersetzen.vi"("Sprachliste"=w378, "String zum Übersetzen"="T90 Test abgeschlossen") -> ("String zum Übersetzen"=w380:string)  [unwired: 9 in, 4 out]
                n129 = call "Strings und Zeitstempel verknuepfen v2.vi"("String 1 hinzufügen"=w380, "Eingangs String"=w376) -> ("Verknüpfter String"=w377:string)  [unwired: 9 in]
              }
            }
          }
        }
      }
      frame "Auswerten" {
        n130 = call "FGV-Funktionstasten.vi"("Herkunft"="T90 Test", "Zustand"=Zustaende."Standby", "Aktion"=Funktionstasten-Aktion."Zustand setzen") -> ()  [unwired: 5 in, 8 out]
        n131 = call "FGV CalGas.vi"("Aktionen"=FGV_CalGas_Aktionen."Aufschaltung CalGas", "Aufschaltung CalGas"=w381) -> ()  [unwired: 5 in, 5 out]
        n132 = call "FGV Datenmanagment.vi"("Aktion"=Aktion_FGV_Datenmanagment."Auswerten") -> ()  [unwired: 7 in, 8 out]
        n133 = call "FGV T90.vi"("Aktion"=Aktion_FGV_T90."T90 inaktiv") -> ()  [unwired: 9 in, 6 out]
      }
      frame "abbrechen" {
        n134 = call "FGV CalGas.vi"("Aktionen"=FGV_CalGas_Aktionen."Aufschaltung CalGas", "Aufschaltung CalGas"=w396) -> ()  [unwired: 5 in, 5 out]
        n135 = call "FGV-Funktionstasten.vi"("Herkunft"="T90 Test", "Zustand"=Zustaende."Standby", "Aktion"=Funktionstasten-Aktion."Zustand setzen") -> ()  [unwired: 5 in, 8 out]
        n136 = call "FGV T90.vi"("Aktion"=Aktion_FGV_T90."T90 inaktiv") -> ()  [unwired: 9 in, 6 out]
        n137 = call "Texte in VIs uebersetzen.vi"("Sprachliste"=w404, "String zum Übersetzen"="T90 Test wurde abgebrochen.") -> ("String zum Übersetzen"=w395:string)  [unwired: 9 in, 4 out]
      }
      frame "Störung" {
        n138 = call "FGV Datenmanagment.vi"("Aktion"=Aktion_FGV_Datenmanagment."init") -> ()  [unwired: 7 in, 8 out]
        n139 = call "FGV CalGas.vi"("Aktionen"=FGV_CalGas_Aktionen."Aufschaltung CalGas", "Aufschaltung CalGas"=w409) -> ()  [unwired: 5 in, 5 out]
        n140 = call "FGV-Funktionstasten.vi"("Herkunft"="T90 Test", "Zustand"=Zustaende."Standby", "Aktion"=Funktionstasten-Aktion."Zustand setzen") -> ()  [unwired: 5 in, 8 out]
        n141 = call "FGV T90.vi"("Aktion"=Aktion_FGV_T90."T90 inaktiv") -> ()  [unwired: 9 in, 6 out]
      }
      frame "fertig" {
      }
    }
  }
  "Status" <- w3
  "Aktion" <- w1
